vi "Open_Doors.vi"(8 "error in (no error)":errorcluster, 10 "Elevator in":T1, 11 "Elevator Fleet in":T8) -> (0 "error out":errorcluster, 2 "Elevator out":T1, 3 "Elevator Fleet out":T8)   [LabVIEW 2026]
uses:
  Controls/Door_Status_Enum.ctl
  Controls/Occupy_Status.ctl
  Controls/Floor_Status.ctl
  Controls/Motion_Status_Enum.ctl
  Controls/Car_Calls_Status.ctl
  Controls/Hall_Calls_Status.ctl
  Controls/Elevator_Status.ctl
  Controls/Elevator_Fleet.ctl
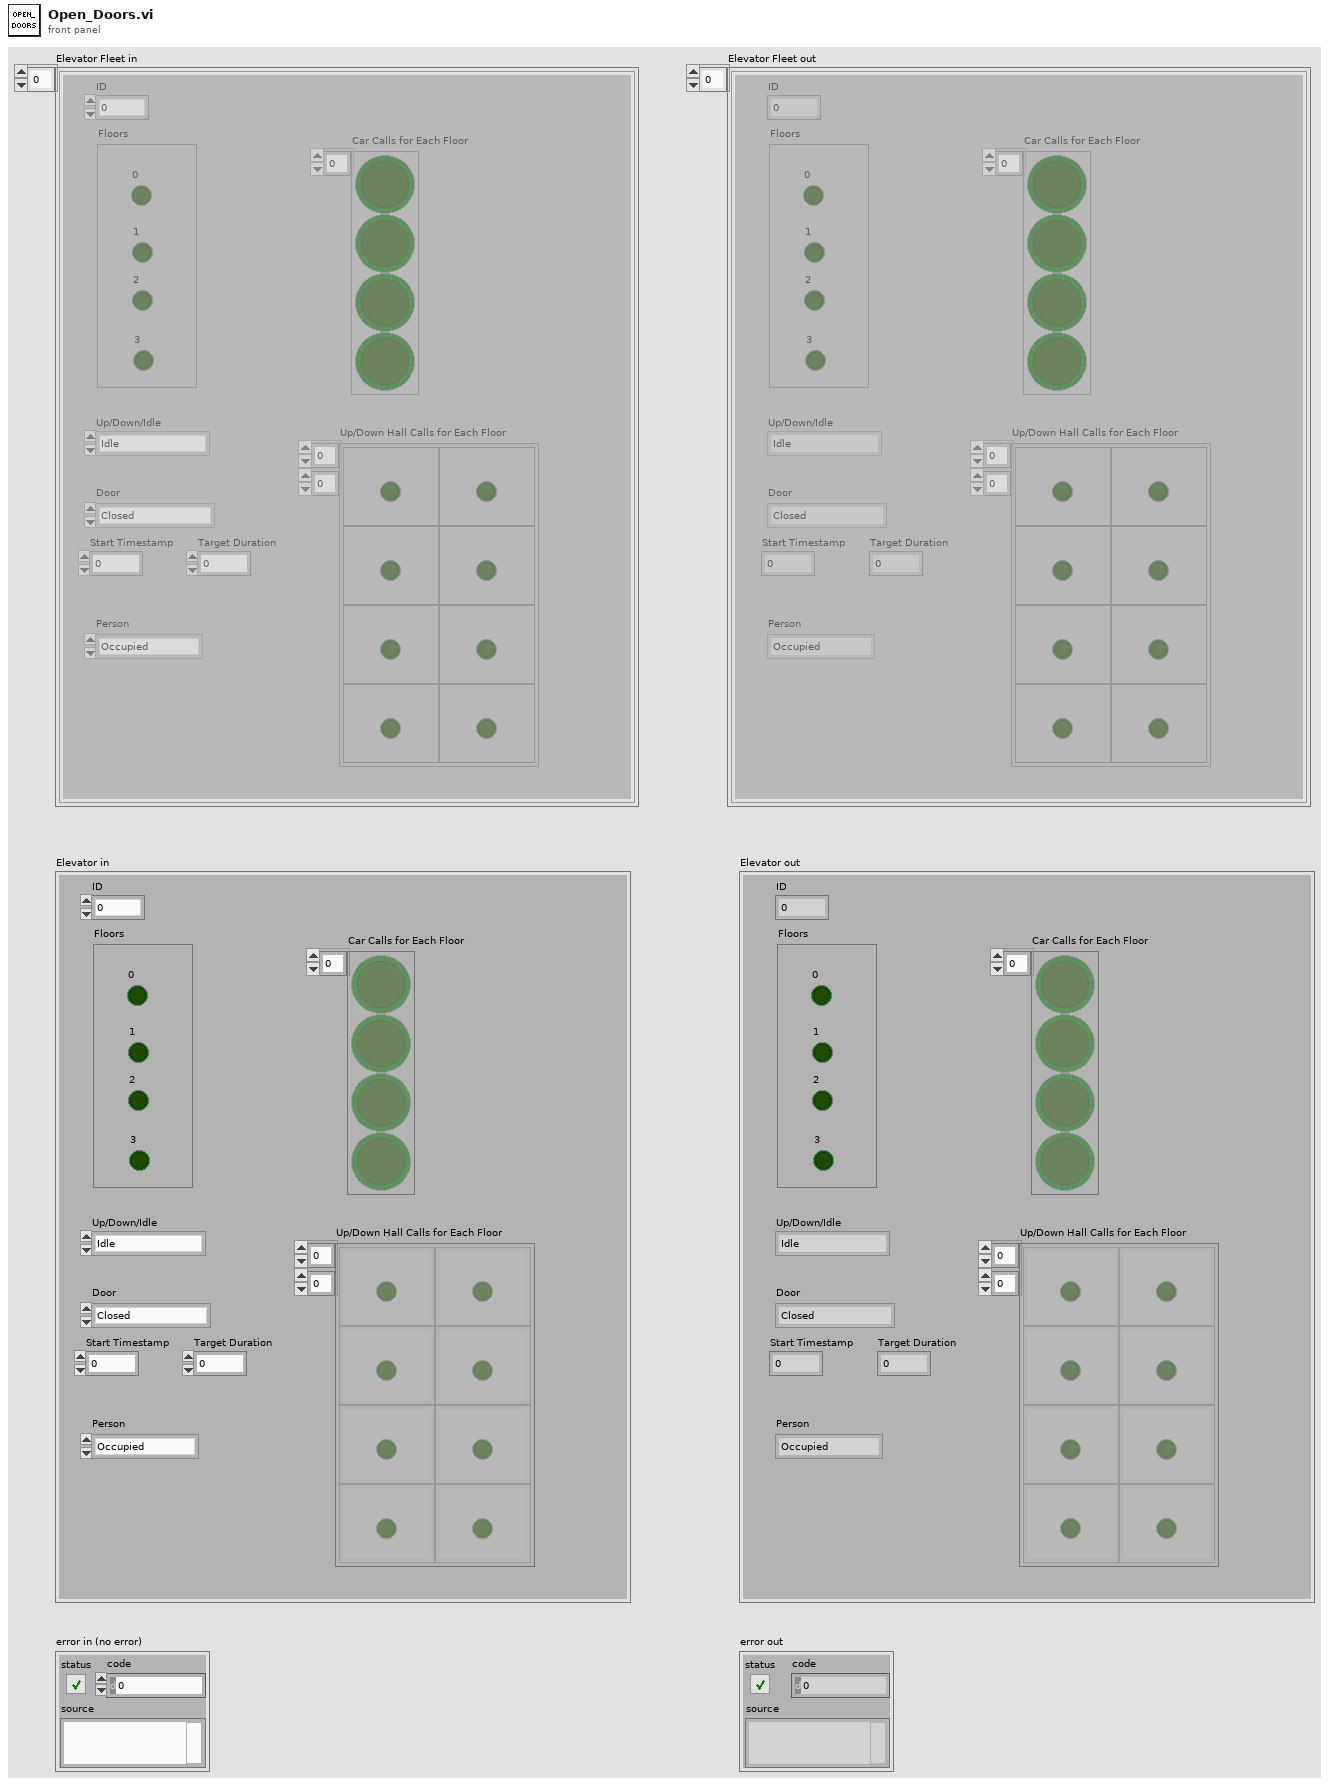
[diagram p1: front panel]
types:
  T1 = typedef "Elevator_Status.ctl" = cluster{"Door":T2, "Person":T3, "Floors":T4, "Up/Down/Idle":T5, "Car Calls for Each Floor":T6, "Up/Down Hall Calls for Each Floor":T7, "ID":i32, "Start Timestamp":u32, "Target Duration":dbl}
  T2 = typedef "Door_Status_Enum.ctl" = enum16{"Closed", "Open", "Opening", "Closing"}
  T3 = typedef "Occupy_Status.ctl" = enum16{"Occupied", "Empty"}
  T4 = typedef "Floor_Status.ctl" = cluster{"0":bool, "1":bool, "2":bool, "3":bool}
  T5 = typedef "Motion_Status_Enum.ctl" = enum16{"Idle", "Up", "Down"}
  T6 = typedef "Car_Calls_Status.ctl" = bool[]
  T7 = typedef "Hall_Calls_Status.ctl" = cluster{bool}[][]
  T8 = typedef "Elevator_Fleet.ctl" = T1[]
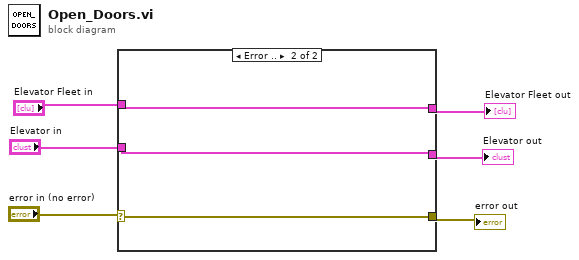
[diagram p0: block diagram]
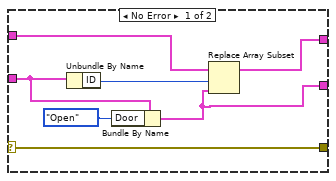
[diagram p2: hidden frame]
diagram:
  n1 = case shown="Error .." "error in (no error)" {
    selector: "error in (no error)" -> [w7 w14]
    tunnel: [w13 w16] -> w6
    tunnel: "Elevator in" -> [w11 w15]
    tunnel: "Elevator Fleet in" -> [w10 w16]
    tunnel: [w8 w15] -> w3
    tunnel: [w7 w14] -> w1
    frame No Error {
      n2 = Unbundle By Name(w11) -> ("ID"=w12:i32)
      n3 = Bundle By Name(cluster=w11, "Door"=Door_Status_Enum."Open") -> (w8:T1)
      n4 = Replace Array Subset(array=w10, new element=w8, index=w12) -> (w13:T8)
    }
    frame Error {
    }
  }
  "Elevator Fleet out" <- w6
  "Elevator out" <- w3
  "error out" <- w1
